vi "attribute_read_double.vi"(5 "Repeated Capability":string, 7 "Attribute":T1={"Identifier"="", "Descriptive name"="", "Data Type"=enum."Integer 32", "Command"="", "Access"=2, "Range Table"="", "Read Callback"="", "Write Callback"="", "Range Callback"="", "Check Callback"="", "Rngtable Callback"="", "Coerce Callback"="", "Supported Models"="", "Instrument Options"="", "Repeated Capabilities"="", "Check Status Callback"="", "Index"=0, "Flag: OPC Wait"=FALSE, "Flag: Dont check status"=FALSE, "Flag: Cache Only"=FALSE} {"Access" items=["Read Only", "Write Only", "Read/Write"]}, 8 "error in":errorcluster, 11 "VISA resource name":refnum<visa-resource-name>) -> (0 "error out":errorcluster, 2 "double out":dbl, 3 "VISA resource name out":refnum<visa-resource-name>)   [LabVIEW 2014, in "rszvl_rsidr_core.lvlib"]
uses:
  rszvl_rsidr_core.lvlib
  type_Attribute.ctl
  type_Attribute_Data_Type.ctl
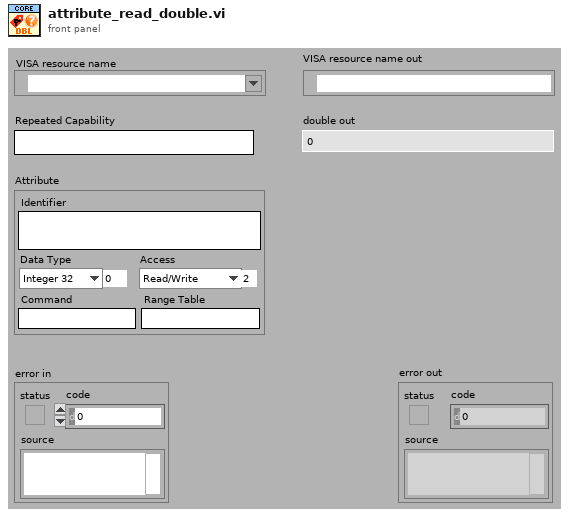
[diagram p1: front panel]
types:
  T1 = typedef "rszvl_rsidr_core.lvlib/type_Attribute.ctl" = cluster{"Identifier":string, "Descriptive name":string, "Data Type":T2, "Command":string, "Access":u16, "Range Table":string, "Read Callback":string, "Write Callback":string, "Range Callback":string, "Check Callback":string, "Rngtable Callback":string, "Coerce Callback":string, "Supported Models":string, "Instrument Options":string, "Repeated Capabilities":string, "Check Status Callback":string, "Index":i32, "Flag: OPC Wait":bool, "Flag: Dont check status":bool, "Flag: Cache Only":bool}
  T2 = typedef "rszvl_rsidr_core.lvlib/type_Attribute_Data_Type.ctl" = enum16{"Integer 32", "Double", "String", "Boolean", "None", "Integer 64"}
  T3 = typedef "rszvl_rsidr_core.lvlib/type_Session_Data.ctl" = cluster{"Instr type":string, "Instr type for err. msg.":string, "Installed Options":string[], "OPC Timeout":i32, "Query Instrument Status":bool, "Check Range":bool, "Check Options":bool, "Add LF to Write":bool, "Simulate":bool, "Logging":bool, "Logging params":variant, "Interface Type":enum16{"Unknown", "GPIB", "VXI", "GPIB_VXI", "ASRL", "PXI", "TCPIP", "USB", "SOCKET"}, "Fast Sweep":i32, "AdditionalFlags":i32, "WaitBeforeWrite":i32, "WaitBeforeRead":i32, "BinDataChunkSize":i64}
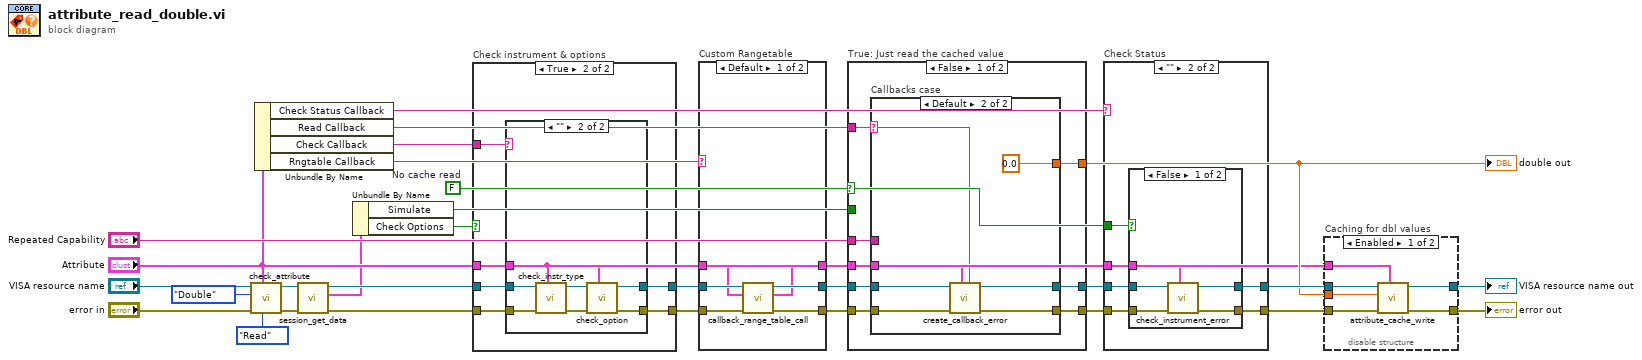
[diagram p0: block diagram]
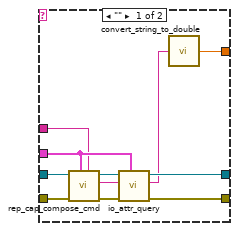
[diagram p2: hidden frame]
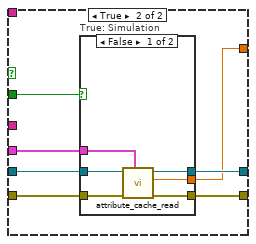
[diagram p3: hidden frame]
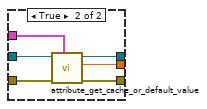
[diagram p4: hidden frame]
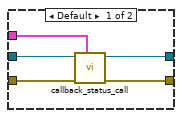
[diagram p6: hidden frame]
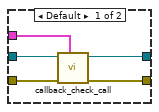
[diagram p9: hidden frame]
diagram:
  w7 = FALSE  # No cache read
  n1 = call "check_attribute.vi"("Access"=enum16{"Read", "Write"}."Read", "Attribute"="Attribute", "error in"="error in", "Data Type"=type_Attribute_Data_Type."Double", "VISA resource name"="VISA resource name") -> ("error out"=w16:errorcluster, "VISA resource name out"=w17:refnum<visa-resource-name>)  [unwired: 5 in]
  n2 = Unbundle By Name("Attribute") -> ("Check Status Callback"=w18:string, "Read Callback"=w19:string, "Check Callback"=w6:string, "Rngtable Callback"=w8:string)
  n3 = call "session_get_data.vi"("error in"=w16, "VISA resource name"=w17) -> ("error out"=w15:errorcluster, "Session User Data out"=w1:T3, "VISA resource name out"=w14:refnum<visa-resource-name>)  [unwired: 7 in]
  n4 = Unbundle By Name(w1) -> ("Simulate"=w2:bool, "Check Options"=w13:bool)
  n5 = case "Check instrument & options" shown="True" w13 {
    tunnel: [w32 w38] -> w12
    tunnel: [w31 w37] -> w11
    tunnel: w6 -> [_ w36]
    tunnel: w15 -> [w31 w35]
    tunnel: w14 -> [w32 w34]
    tunnel: "Attribute" -> [_ w33]
    frame False {
    }
    frame True {
      n6 = case shown="\"\"" w36 {
        tunnel: [w42 w48] -> w38
        tunnel: [w40 w47] -> w37
        tunnel: w35 -> [w41 w46]
        tunnel: w34 -> [w43 w45]
        tunnel: w33 -> [w39 w44]
        frame Default {
          n7 = call "callback_check_call.vi"("Attribute"=w39, "error in"=w41, "VISA resource name"=w43) -> ("error out"=w40:errorcluster, "VISA resource name out"=w42:refnum<visa-resource-name>)  [unwired: 7 in]
        }
        frame "" {
          n8 = call "check_instr_type.vi"("Attribute"=w44, "error in"=w46, "VISA resource name"=w45) -> ("error out"=w50:errorcluster, "VISA resource name out"=w49:refnum<visa-resource-name>)  [unwired: 6 in, 1 out]
          n9 = call "check_option.vi"("Attribute"=w44, "error in"=w50, "VISA resource name"=w49) -> ("error out"=w47:errorcluster, "VISA resource name out"=w48:refnum<visa-resource-name>)  [unwired: 7 in]
        }
      }
    }
  }
  n10 = case "Custom Rangetable" shown="Default" w8 {
    tunnel: w12 -> [w56 w59]
    tunnel: w11 -> [w53 w58]
    tunnel: [w55 w59] -> w10
    tunnel: [w54 w58] -> w9
    tunnel: "Attribute" -> [w52 w57]
    tunnel: [w51 w57] -> w5
    frame Default {
      n11 = call "callback_range_table_call.vi"("error in"=w53, "Attribute in"=w52, "VISA resource name"=w56) -> ("error out"=w54:errorcluster, "Attribute out"=w51:T1, "VISA resource name out"=w55:refnum<visa-resource-name>)  [unwired: 6 in]
    }
    frame "" {
    }
  }
  n12 = case "True: Just read the cached value" shown="False" w7 {
    tunnel: "Repeated Capability" -> [w67 _]
    tunnel: [w66 w89] -> w21
    tunnel: [w65 w90] -> w20
    tunnel: [w64 w88] -> w26
    tunnel: w19 -> [w63 _]
    tunnel: w10 -> [w62 w92]
    tunnel: w9 -> [w61 w91]
    tunnel: w5 -> [w60 w87]
    tunnel: w2 -> [_ w86]
    frame False {
      n13 = case "Callbacks case" shown="Default" w63 {
        selector: w63 -> [_ w80]
        tunnel: w62 -> [w78 w84]
        tunnel: w61 -> [w77 w85]
        tunnel: w67 -> [w70 _]
        tunnel: [w75 w82] -> w65
        tunnel: [w68 w83] -> w66
        tunnel: [w76 0.0 ("Attribute Value Double")] -> w64
        tunnel: w60 -> [w71 w81]
        frame "" {
          n14 = call "rep_cap_compose_cmd.vi"("Repeated Capability"=w70, "Attribute"=w71, "error in"=w77, "VISA resource name"=w78) -> ("error out"=w74:errorcluster, "Command out"=w73:string, "VISA resource name out"=w72:refnum<visa-resource-name>)  [unwired: 5 in]
          n15 = call "io_attr_query.vi"("Attribute"=w71, "error in"=w74, "write buffer"=w73, "VISA resource name"=w72) -> ("error out"=w68:errorcluster, "read buffer"=w69:string, "VISA resource name out"=w75:refnum<visa-resource-name>)  [unwired: 5 in]
          n16 = call "convert_string_to_double.vi"("String in"=w69) -> ("double value out"=w76:dbl)  [unwired: 4 in]
        }
        frame Default {
          n17 = call "create_callback_error.vi"("Callback Name"=w80, "Attribute"=w81, "error in"=w85, "VISA resource name"=w84) -> ("error out"=w83:errorcluster, "VISA resource name out"=w82:refnum<visa-resource-name>)  [unwired: 6 in]
        }
      }
    }
    frame True {
      n18 = case "True: Simulation" shown="False" w86 {
        tunnel: w91 -> [w98 w104]
        tunnel: w92 -> [w97 w103]
        tunnel: w87 -> [w96 w100]
        tunnel: [w95 w102] -> w89
        tunnel: [w94 w101] -> w90
        tunnel: [w93 w99] -> w88
        frame False {
          n19 = call "attribute_cache_read.vi"("Attribute"=w96, "error in"=w98, "VISA resource name"=w97) -> ("error out"=w95:errorcluster, "Double out"=w93:dbl, "VISA resource name out"=w94:refnum<visa-resource-name>)  [unwired: 1 in, 5 out]
        }
        frame True {
          n20 = call "attribute_get_cache_or_default_value.vi"("Attribute"=w100, "error in"=w104, "VISA resource name"=w103) -> ("error out"=w102:errorcluster, "Double out"=w99:dbl, "VISA resource name out"=w101:refnum<visa-resource-name>)  [unwired: 1 in, 5 out]
        }
      }
    }
  }
  "double out" <- w26
  n21 = case "Check Status" shown="\"\"" w18 {
    tunnel: w21 -> [w109 w113]
    tunnel: [w108 w112] -> w27
    tunnel: [w107 w114] -> w28
    tunnel: w20 -> [w106 w115]
    tunnel: w5 -> [w105 w111]
    tunnel: w7 -> [_ w110]
    frame Default {
      n22 = call "callback_status_call.vi"("Attribute"=w105, "error in"=w109, "VISA resource name"=w106) -> ("error out"=w108:errorcluster, "VISA resource name out"=w107:refnum<visa-resource-name>)  [unwired: 7 in]
    }
    frame "" {
      n23 = case shown="False" w110 {
        tunnel: w115 -> [w120 w122]
        tunnel: [w119 w122] -> w114
        tunnel: w113 -> [w118 w121]
        tunnel: [w117 w121] -> w112
        tunnel: w111 -> [w116 _]
        frame False {
          n24 = call "check_instrument_error.vi"("Attribute"=w116, "error in"=w118, "VISA resource name"=w120) -> ("error out"=w117:errorcluster, "VISA resource name out"=w119:refnum<visa-resource-name>)  [unwired: 7 in]
        }
        frame True {
        }
      }
    }
  }
  n25 = disable-structure "Caching for dbl values" shown="Enabled" {
    disable-tunnel: [w128 w130] -> w23
    disable-tunnel: [w127 w129] -> w24
    disable-tunnel: w27 -> [w126 w129]
    disable-tunnel: w28 -> [w125 w130]
    disable-tunnel: w26 -> [w124 _]
    disable-tunnel: "Attribute" -> [w123 _]
    frame Enabled {
      n26 = call "attribute_cache_write.vi"("Attribute"=w123, "error in"=w126, "Value in"=w124, "VISA resource name"=w125) -> ("error out"=w127:errorcluster, "VISA resource name out"=w128:refnum<visa-resource-name>)  [unwired: 6 in]
    }
    frame Disabled {
    }
  }
  "error out" <- w24
  "VISA resource name out" <- w23
